vi "GetSystemCfg.vi"(0 "SystemCfg":string(combo), 5 "error in (no error)":errorcluster caption="错误输入（无错误）") -> (14 "Ini File Path":path, 19 "error out":errorcluster caption="错误输出")   [LabVIEW 2013]
uses:
  <vilib>/Utility/config.llb/Read Key (String).vi
  <vilib>/Utility/config.llb/NI_LVConfig.lvlib
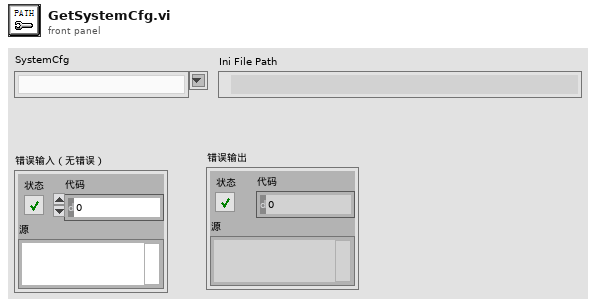
[diagram p1: front panel]
types:
  T1 = typedef "NI_LVConfig.lvlib/Config Data RefNum.ctl" = refnum<k1>
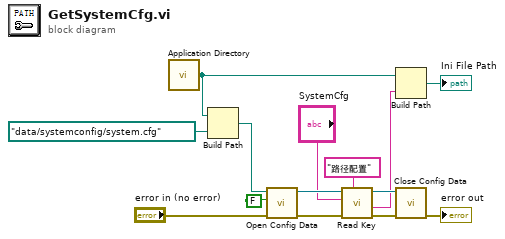
[diagram p0: block diagram]
diagram:
  n1 = call <vilib>:"Application Directory.vi"() -> ("Application Directory"=w4:path)
  n2 = Build Path(base path=w4, name or relative path=path "data/systemconfig/system.cfg") -> (appended path=w7:path)
  n3 = call <vilib>:"Open Config Data.vi"("error in (no error)"="error in (no error)", "create file if necessary (T)"=FALSE, "configuration file path"=w7) -> ("error out"=w11:errorcluster, "refnum"=w5:T1)  [unwired: 6 in, 1 out]
  n4 = call-poly <vilib>:"Read Key.vi"("section"="路径配置" ("key"), "error in (no error)"=w11, "key"="SystemCfg", "refnum"=w5) -> ("error out"=w8:errorcluster, "value"=w3:string, "refnum out"=w9:T1)  [unwired: 4 in, 1 out]
  n5 = Build Path(base path=w4, name or relative path=w3) -> (appended path=→"Ini File Path":path)
  n6 = call <vilib>:"Close Config Data.vi"("error in (no error)"=w8, "refnum"=w9) -> ("error out"=→"error out":errorcluster)  [unwired: 8 in, 1 out]
